vi "Driver Update.vi"(8 "error in (no error)":errorcluster, 10 "Driver Record":T2, 11 "Connection Refnum":T1) -> (0 "error out":errorcluster, 3 "Connection Refnum":T1)   [LabVIEW 2011]
uses:
  Driver Record.ctl
  Summitek EXT/ODBC/SQL Controls/Connection Refnum.ctl
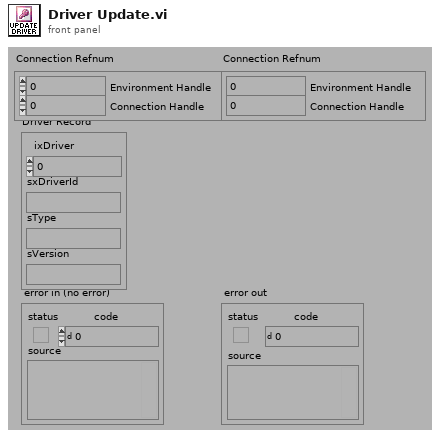
[diagram p1: front panel]
types:
  T1 = typedef "Connection Refnum.ctl" = cluster{"Environment Handle":i32, "Connection Handle":i32}
  T2 = typedef "Driver Record.ctl" = cluster{"ixDriver":i32, "sxDriverId":string, "sType":string, "sVersion":string}
  T3 = typedef "Statement Refnum.ctl" = cluster{"Statement Handle":i32, "Parameter Number":u16}
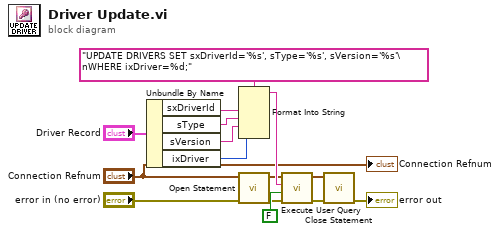
[diagram p0: block diagram]
diagram:
  n1 = Unbundle By Name("Driver Record") -> ("sxDriverId"=w9:string, "sType"=w8:string, "sVersion"=w5:string, "ixDriver"=w4:i32)
  n2 = Format Into String(format string="UPDATE DRIVERS SET sxDriverId='%s', sType='%s', sVersion='%s'\nWHERE ixDriver=%d;" ("User Query"), w9, w8, w5, w4) -> (resulting string=w10:string)  [unwired: 2 in, 1 out]
  n3 = call "Open Statement.vi"("error in (no error)"="error in (no error)", "Connection Refnum"="Connection Refnum") -> ("error out"=w7:errorcluster, "Statement Refnum"=w6:T3)  [unwired: 4 out]
  n4 = call "Execute User Query.vi"("error in (no error)"=w7, "Return Data? (f)"=FALSE, "User Query"=w10, "Statement Refnum"=w6) -> ("error out"=w13:errorcluster, "Statement Refnum"=w12:T3)  [unwired: 2 out]
  n5 = call "Close Statement.vi"("error in (no error)"=w13, "Statement Refnum"=w12) -> ("error out"=→"error out":errorcluster)  [unwired: 5 out]
  "Connection Refnum" <- "Connection Refnum"
